vi "Main.vi"(0 "VI to load":string(combo)="Latch boolean simulation", 5 "STOP":bool, 11 "Error In":errorcluster) -> (15 "Error Out":errorcluster)   [LabVIEW 2016, in "Subpanel.lvlib"]
doc: "Source VI to test subpanel"
uses:
  Subpanel.lvlib
  NumericControlValueCoercion.vi
  BooleanControl.vi
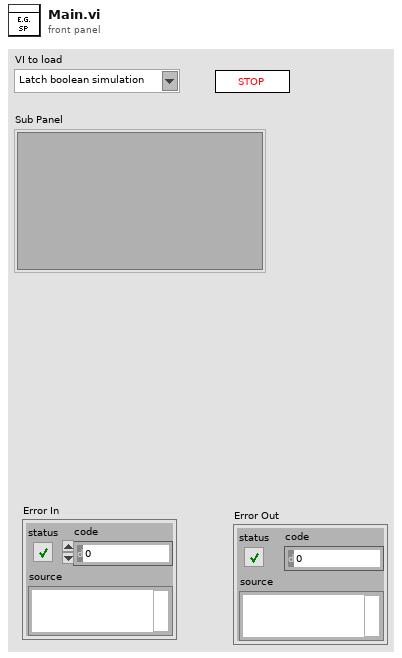
[diagram p1: front panel]
types:
  T1 = enum32{"Invalid", "Standard", "Closed", "Hidden", "Minimized", "Maximized"}
  T2 = enum32{"invalid app kind", "Development System", "Run Time System", "Student Edition", "Embedded LabVIEW", "Evaluation", "Custom"}
  T3 = cluster{"Core":cluster{"Current VI Reference":refnum<vi>, "Close Panel on Exit?":bool}, "Data Cluster":cluster{"Flags":cluster{"Source Code?":bool, "VI Inserted?":bool}, "VI Details":string[], "VI Ref[]":refnum<vi>[], "VI Ref":refnum<vi>}}
  T4 = cluster{"Flags":cluster{"Source Code?":bool, "VI Inserted?":bool}, "VI Details":string[], "VI Ref[]":refnum<vi>[], "VI Ref":refnum<vi>}
  T5 = cluster{"Current VI Reference":refnum<vi>, "Close Panel on Exit?":bool}
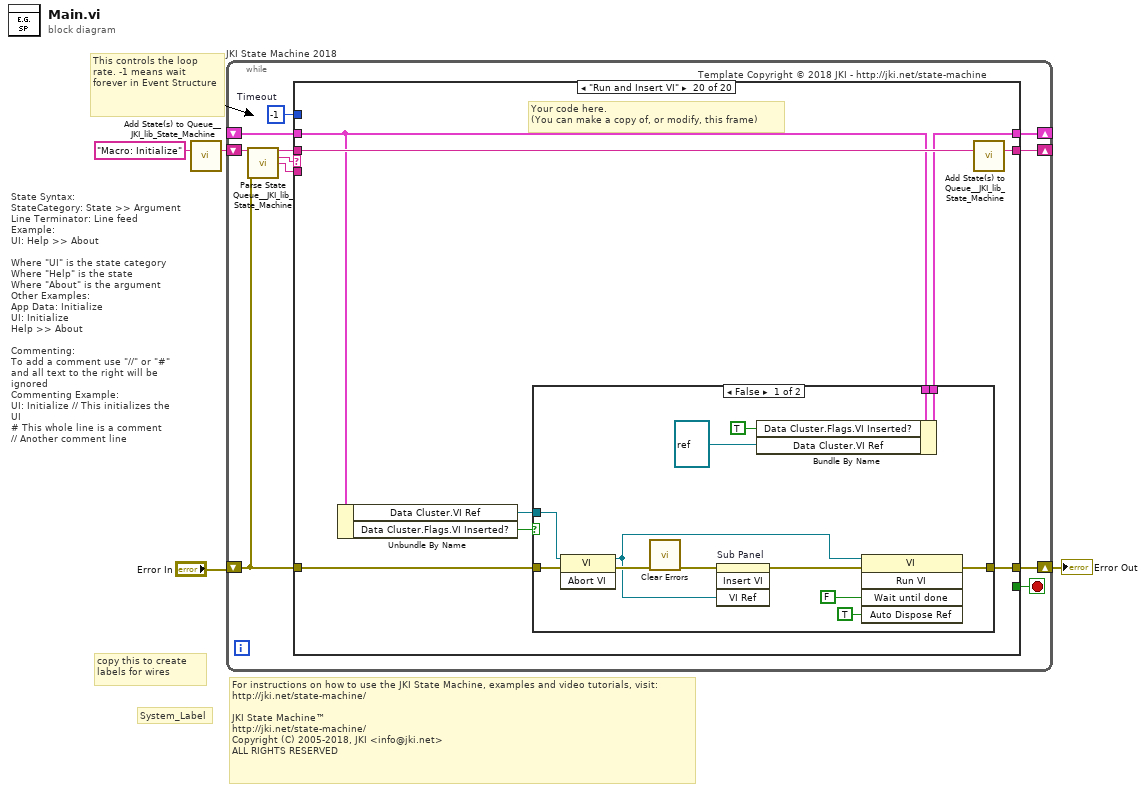
[diagram p0: block diagram]
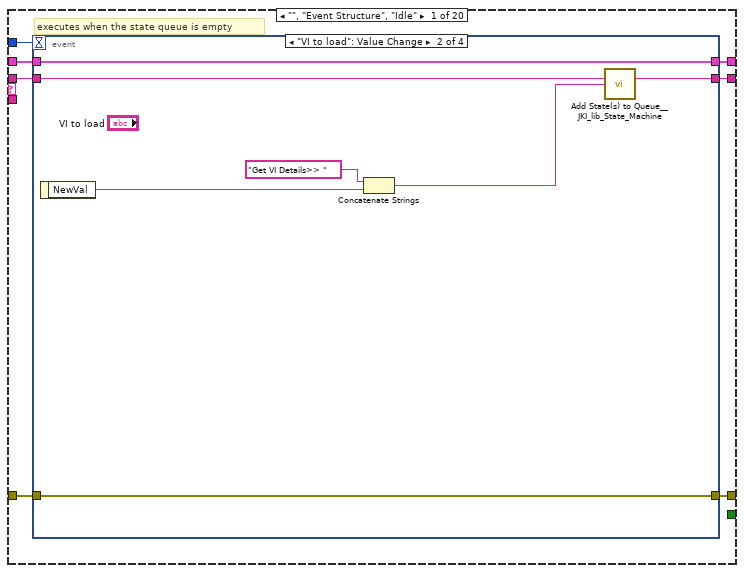
[diagram p2: hidden frame]
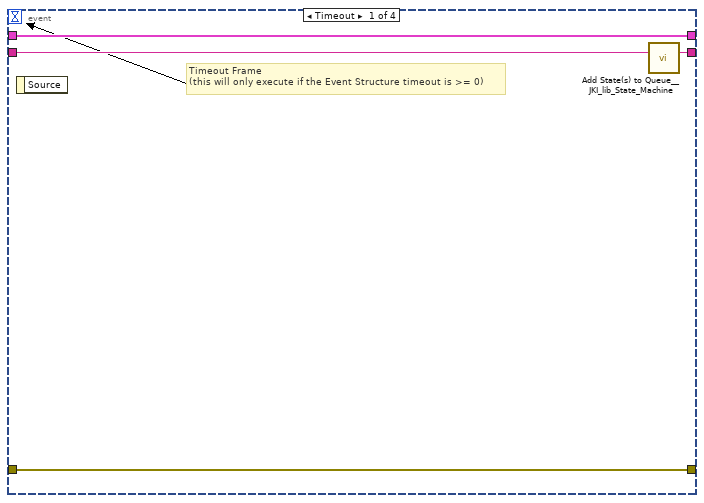
[diagram p3: hidden frame]
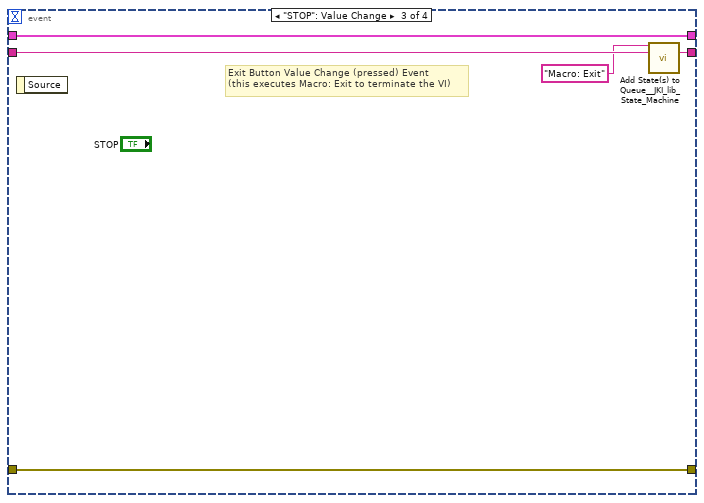
[diagram p4: hidden frame]
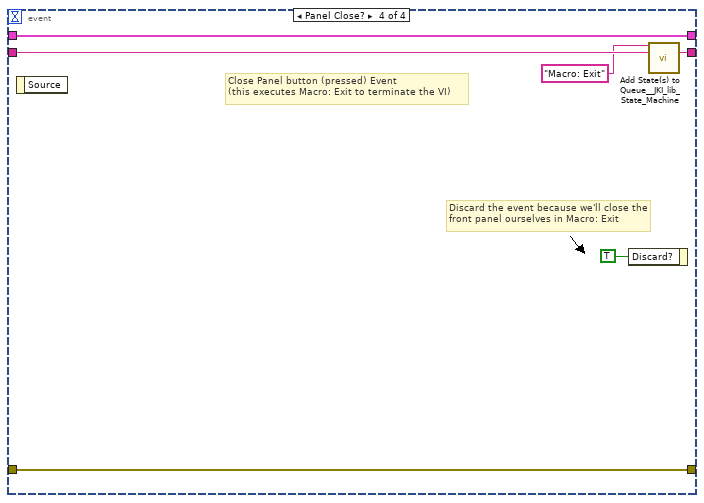
[diagram p5: hidden frame]
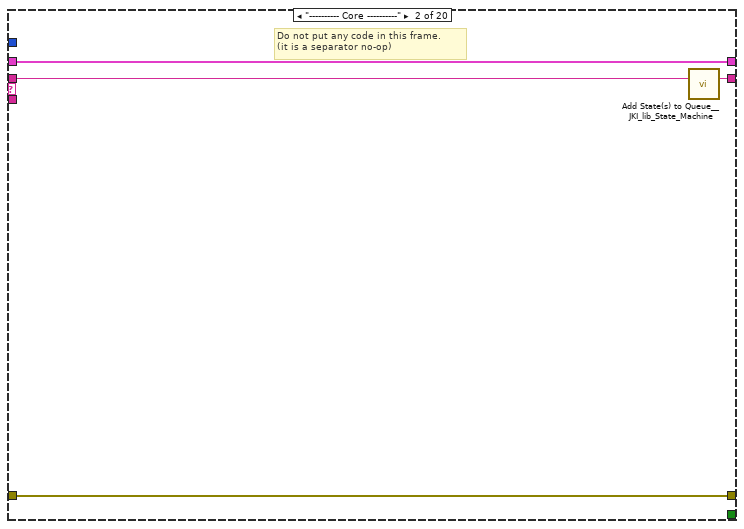
[diagram p6: hidden frame]
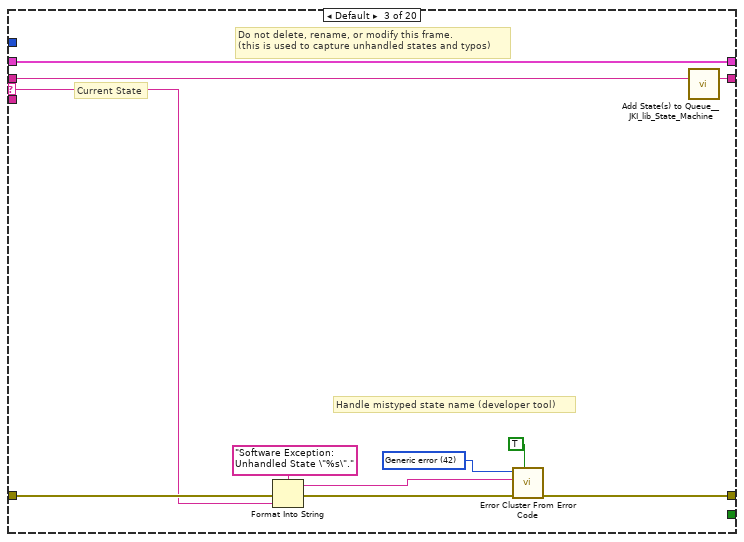
[diagram p7: hidden frame]
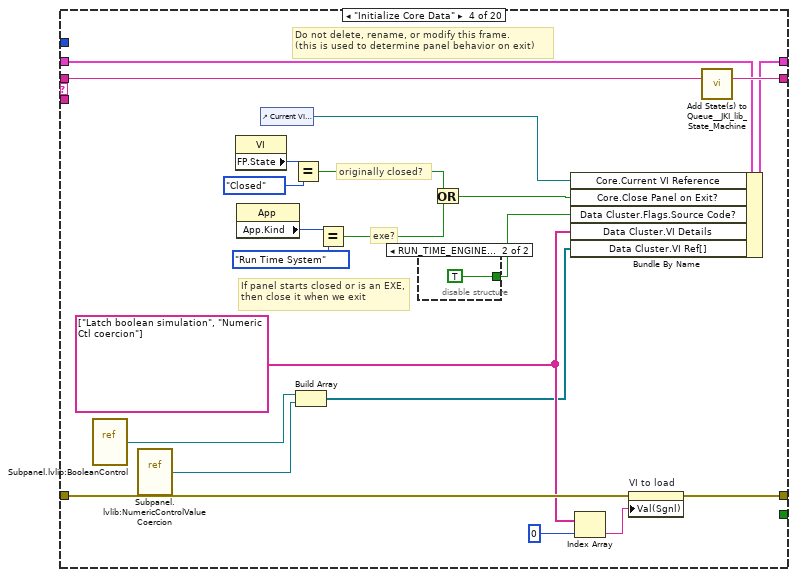
[diagram p8: hidden frame]
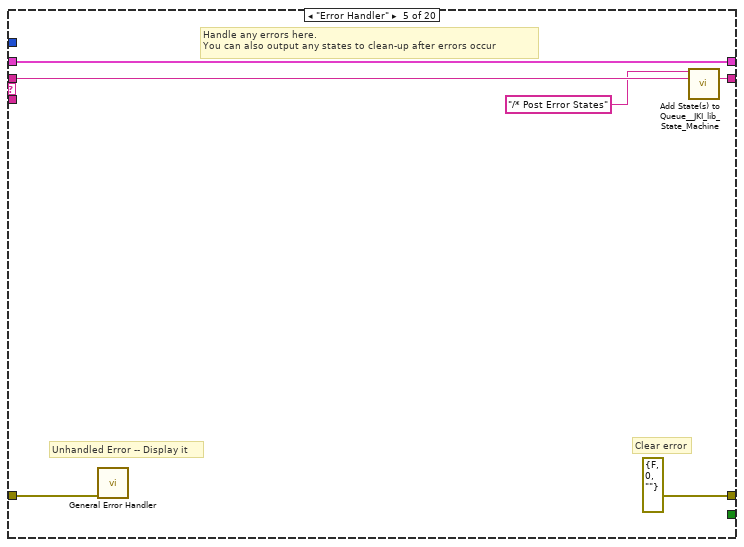
[diagram p10: hidden frame]
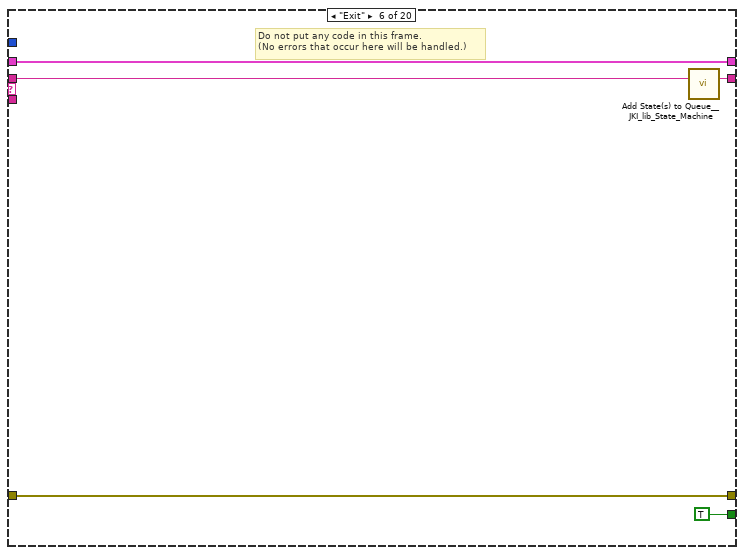
[diagram p11: hidden frame]
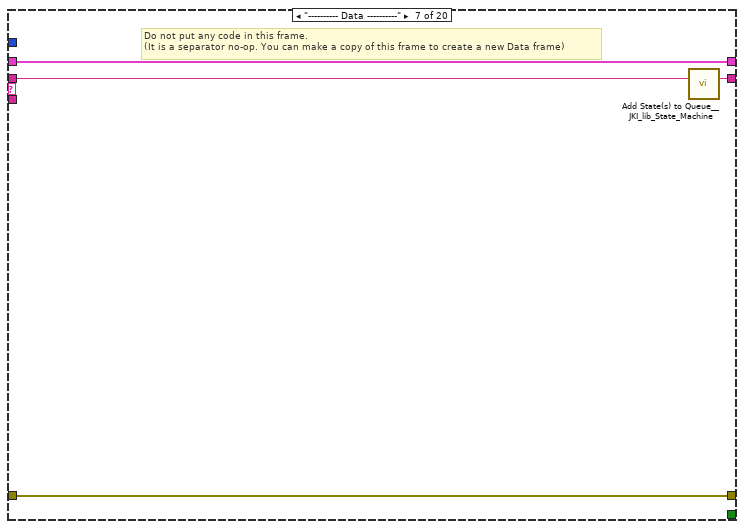
[diagram p12: hidden frame]
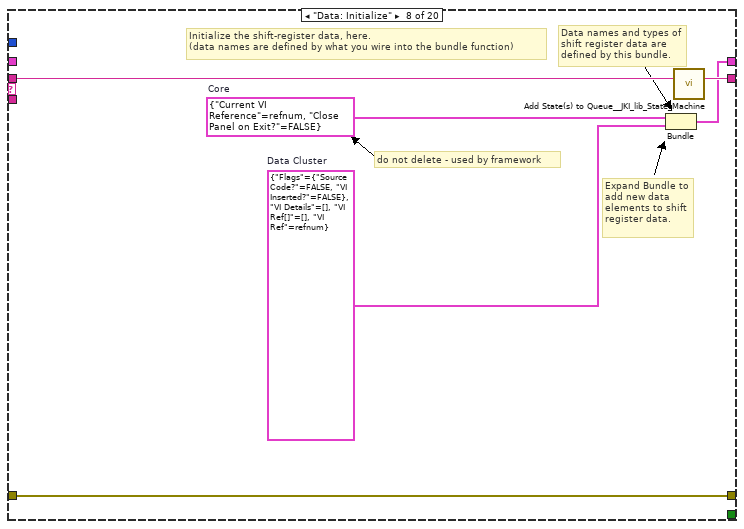
[diagram p13: hidden frame]
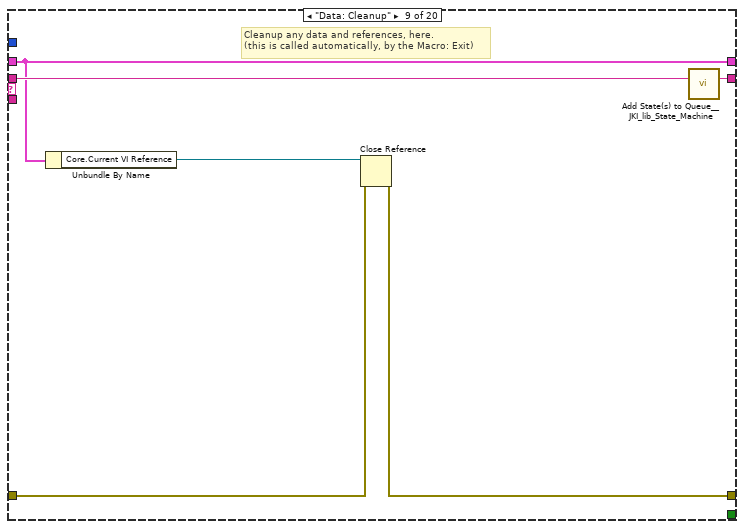
[diagram p14: hidden frame]
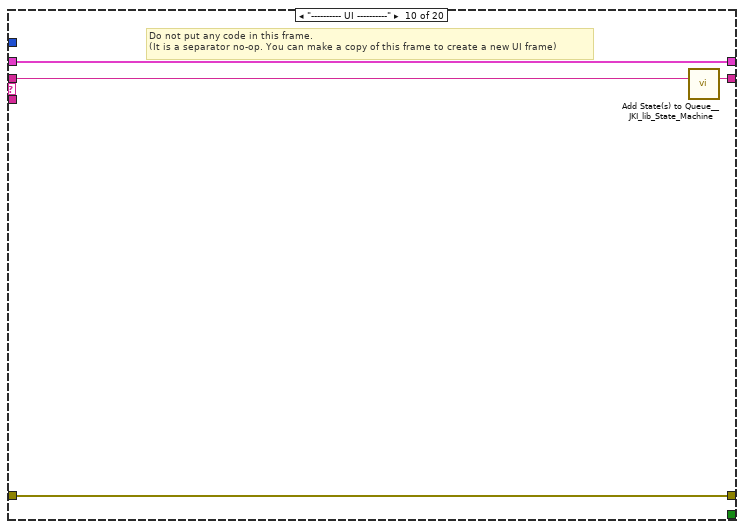
[diagram p15: hidden frame]
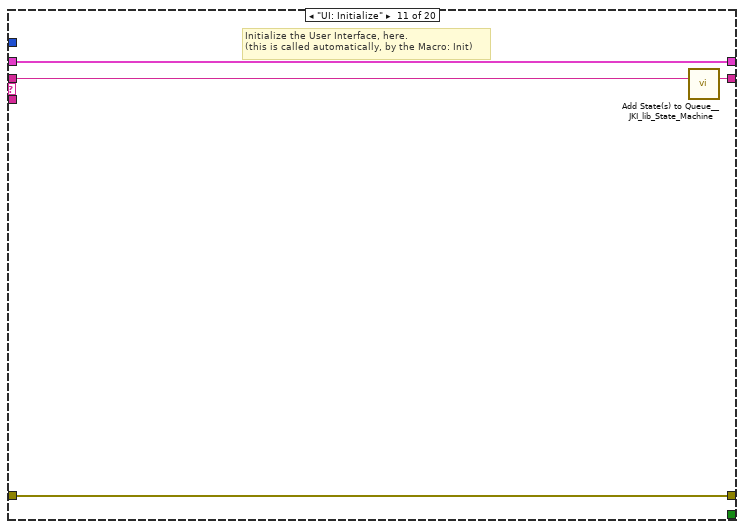
[diagram p16: hidden frame]
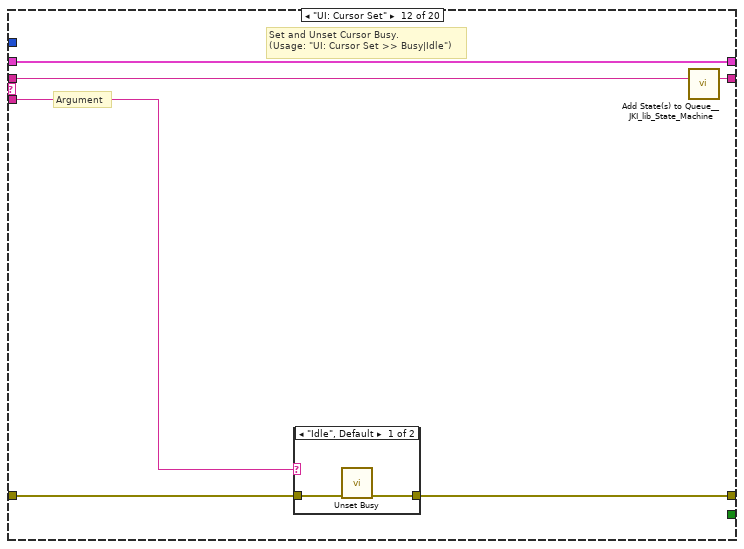
[diagram p17: hidden frame]
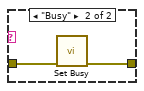
[diagram p18: hidden frame]
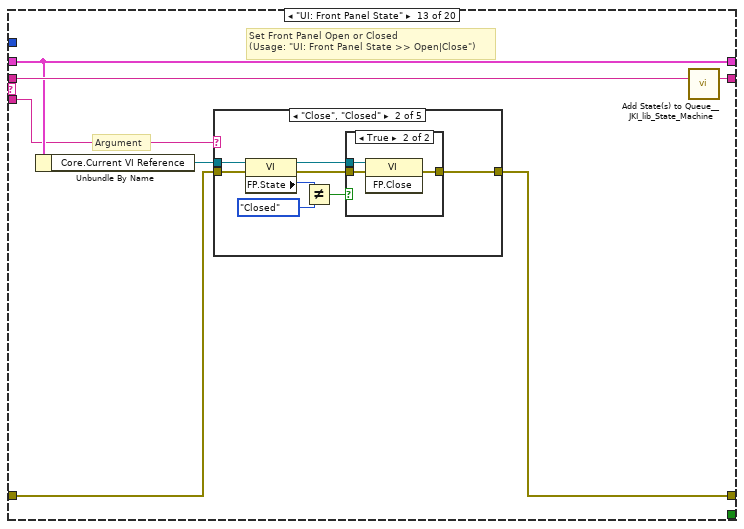
[diagram p19: hidden frame]
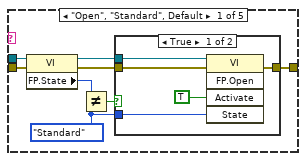
[diagram p20: hidden frame]
diagram:
  # "For instructions on how to use the JKI State Machine, examples and video tutorials, visit:\nhttp://jki.net/state-machine/\n\nJKI State Machine™\nhttp://jki.net/state-machine/\nCopyright (C) 2005-2018, JKI <info@jki.net>\nALL RIGHTS RESERVED"
  # "State Syntax:\nStateCategory: State >> Argument\nLine Terminator: Line feed\nExample:\nUI: Help >> About\n\nWhere \"UI\" is the state category\nWhere \"Help\" is the state\nWhere \"About\" is the argument\nOther Examples:\nApp Data: Initialize\nUI: Initialize\nHelp >> About\n\nCommenting:\nTo add a comment use \"//\" or \"#\" and all text to the right will be ignored\nCommenting Example:\nUI: Initialize // This initializes the UI\n# This whole line is a comment\n// Another comment line"
  # "copy this to create labels for wires"
  # "This controls the loop rate. -1 means wait forever in Event Structure"
  # "System_Label"
  n1 = call <vilib>:"Add State(s) to Queue__JKI_lib_State_Machine.vi"("State(s) in (\"\")"="Macro: Initialize") -> ("States Out"=w4:string)  [unwired: 14 in]
  n2 = while "JKI State Machine 2018" {
    shift-right: [w8] -> _
    shift-left: _ -> [w7]
    shift-right: [w11] -> w2
    shift-left: "Error In" -> [w5]
    shift-right: [w10] -> _
    shift-left: w4 -> [w12]
    stop <- w9 stop-if-true
    w6 = -1  # Timeout
    # "Template Copyright © 2018 JKI - http://jki.net/state-machine"
    n3 = call <vilib>:"Parse State Queue__JKI_lib_State_Machine.vi"("State Queue"=w12, "Error In (no error)"=w5) -> ("Remaining States"=w14:string, "Current State"=w15:string, "Arguments"=w13:string)  [unwired: 11 in]
    n4 = case shown="\"Run and Insert VI\"" w15 {
      selector: w15 -> [_ _ w49 _ _ _ _ _ _ _ _ _ _ _ _ _ _ _ _ _]
      tunnel: w14 -> [w22 w48 w53 w80 w87 w92 w96 w102 w108 w112 w116 w122 w133 w202 w207 w217 w221 w232 w240 w260]
      tunnel: w13 -> [_ _ _ _ _ _ _ _ _ _ _ w117 w127 _ _ _ _ w229 _ _]
      tunnel: w7 -> [w20 w45 w51 w73 w84 w90 w93 _ w103 w109 w114 w120 w129 w199 w204 w214 w218 w227 w234 w253]
      tunnel: [w19 w46 w55 w66 errorcluster {"status"=FALSE, "code"=0, "source"=""} ("error out") w89 w94 w99 w104 w110 w113 w118 w130 w200 w205 w215 w219 w223 w235 w255] -> w11
      tunnel: w5 -> [w18 w46 w54 w77 w83 w89 w94 w99 w105 w110 w113 w119 w131 w200 w205 w215 w219 w223 w236 w256]
      tunnel: [w21 w47 w52 w79 w86 w91 w95 w101 w107 w111 w115 w121 w132 w201 w206 w216 w220 w231 w239 w259] -> w10
      tunnel: [_ _ _ _ _ TRUE _ _ _ _ _ _ _ _ _ _ _ _ _ _] -> w9
      tunnel: [w17 w45 w51 w78 w84 w90 w93 w100 w103 w109 w114 w120 w129 w199 w204 w214 w218 w226 w233 w254] -> w8
      tunnel: w6 -> [w16 _ _ _ _ _ _ _ _ _ _ _ _ _ _ _ _ _ _ _]
      frame "", "Event Structure", "Idle" {
        # "executes when the state queue is empty"
        n5 = event shown="[1] \"VI to load\": Value Change" {
          selector: _ -> [_ _ _ _]
          dyn-events: _ -> [_ _ _ _]
          timeout: w16 -> [_ _ _ _]
          tunnel: w22 -> [w26 w33 w38 w44]
          tunnel: [w25 w32 w37 w43] -> w21
          tunnel: w20 -> [w23 w31 w35 w41]
          tunnel: [w24 w27 w36 w42] -> w19
          tunnel: w18 -> [w24 w27 w36 w42]
          tunnel: [w23 w31 w35 w41] -> w17
          event Timeout {
            # "Timeout Frame\n(this will only execute if the Event Structure timeout is >= 0)"
            n6 = event-data() -> ()  [unwired: 1 in, 1 out]
            n7 = call <vilib>:"Add State(s) to Queue__JKI_lib_State_Machine.vi"("State(s) in (\"\")"=w26) -> ("States Out"=w25:string)  [unwired: 14 in]
          }
          event "VI to load": Value Change {
            n8 = event-data() -> ("NewVal"=w30:string)  [unwired: 1 in]
            n9 = Concatenate Strings("Get VI Details>> " ("Item to Add"), w30) -> (w28:string)
            n10 = call <vilib>:"Add State(s) to Queue__JKI_lib_State_Machine.vi"("State(s) in (\"\")"=w33, "State(s) at Back (\"\")"=w28) -> ("States Out"=w32:string)  [unwired: 13 in]
          }
          event "STOP": Value Change {
            # "Exit Button Value Change (pressed) Event\n(this executes Macro: Exit to terminate the VI)"
            n11 = event-data() -> ()  [unwired: 1 in, 1 out]
            n12 = call <vilib>:"Add State(s) to Queue__JKI_lib_State_Machine.vi"("State(s) in Front (\"\")"="Macro: Exit", "State(s) in (\"\")"=w38) -> ("States Out"=w37:string)  [unwired: 13 in]
          }
          event Panel Close? {
            # "Discard the event because we'll close the front panel ourselves in Macro: Exit"
            # "Close Panel button (pressed) Event\n(this executes Macro: Exit to terminate the VI)"
            n13 = event-data() -> ()  [unwired: 1 in, 1 out]
            n14 = event-data("Discard?"=TRUE) -> ()  [unwired: 1 in, 1 out]
            n15 = call <vilib>:"Add State(s) to Queue__JKI_lib_State_Machine.vi"("State(s) in Front (\"\")"="Macro: Exit", "State(s) in (\"\")"=w44) -> ("States Out"=w43:string)  [unwired: 13 in]
          }
        }
      }
      frame "---------- Core ----------" {
        # "Do not put any code in this frame.\n(it is a separator no-op)"
        n16 = call <vilib>:"Add State(s) to Queue__JKI_lib_State_Machine.vi"("State(s) in (\"\")"=w48) -> ("States Out"=w47:string)  [unwired: 14 in]
      }
      frame Default {
        w58 = 42 items=["No error", "Argument error", "Memory is full", "Out of zone", "End of file", "File already open", "Generic file I/O error", "File not found", "File permission error", "Disk is full", "Duplicate path", "Too many files open", "System feature not enabled", "Resource file not found", "Cannot add resource", "Resource not found", "Image not found", "Image memory error", "Pen does not exist", "Config type invalid", "Config token not found", "Config parse error", "Config memory error", "Bad external code format", "Bad external code offset", "External code not present", "Null window", "Destroy window error", "Null menu", "Print aborted", "Bad print record", "Print driver error", "Windows error during printing", "Memory error during printing", "Print dialog error", "Generic print error", "Invalid device refnum", "Device not found", "Device parameter error", "Device unit error", "Cannot open device", "Device call aborted", "Generic error", "Cancelled by user", "Object ID too low", "Object ID too high", "Object not in heap", "Unknown heap", "Unknown object (invalid DefProc)", "Unknown object (DefProc not in table)", "Message out of range", "Invalid (null) method", "Unknown message", "Manager call not supported", "Bad address", "Network operation in progress", "Network operation timed out", "Connection is busy", "Network attribute not supported", "Network error", "Address in use", "System out of memory", "Connection aborted", "Connection refused", "Not connected", "Already connected", "Connection closed", "Initialization error (interapplication manager)", "Bad occurrence", "Wait on unbound occurrence handler", "Occurrence queue overflow", "Datalog type conflict", "Unused", "Unrecognized type (interapplication manager)", "Memory corrupt", "Failed to make temporary DLL", "Old CIN version", "Drag socket not found", "Failed to load drop-object", "Failed to register OLE object", "Failed to release OLE object", "Format specifier type mismatch", "Unknown format specifier", "Too few format specifiers", "Too many format specifiers", "Scan failed", "Newer CIN version", "Error converting to variant", "Runtime menu error", "Password tampered", "Variant attribute not found", "Incompatible variant data type", "Event data is not available", "Event Store is not present", "Occurrence is not found", "Event Queue is not created", "Event info is not available", "Refnum passed is NULL", "Error retrieving Class GUID", "Error retrieving CoClass GUID", "Error retrieving TypeLib GUID.", "Bad built application magic bytes.", "Specific driver is different from the specific driver associated with the Logical Name.", "There is no session opened to the class driver.", "Max Error", "MAX - Error with config objects", "MAX - Error loading configuration", "MAX - Group not supported"]
        # "Current State"
        # "Do not delete, rename, or modify this frame.\n(this is used to capture unhandled states and typos)"
        # "Handle mistyped state name (developer tool)"
        n17 = Format Into String(format string="Software Exception: Unhandled State \"%s\"." ("message"), error in=w54, w49) -> (resulting string=w57:string, error out=w56:errorcluster)  [unwired: 1 in]
        n18 = call <vilib>:"Error Cluster From Error Code.vi"("show call chain? (False)"=TRUE, "error in (no error)"=w56, "error message (\"\")"=w57, "error code (0)"=w58) -> ("error out"=w55:errorcluster)  [unwired: 5 in]
        n19 = call <vilib>:"Add State(s) to Queue__JKI_lib_State_Machine.vi"("State(s) in (\"\")"=w53) -> ("States Out"=w52:string)  [unwired: 14 in]
      }
      frame "Initialize Core Data" {
        w65 = string[] ["Latch boolean simulation", "Numeric Ctl coercion"]
        # "Do not delete, rename, or modify this frame.\n(this is used to determine panel behavior on exit)"
        # "originally closed?"
        # "exe?"
        # "If panel starts closed or is an EXE, then close it when we exit"
        n20 = vi-ref "Subpanel.lvlib:BooleanControl.vi"() -> (w61:refnum<vi>)
        n21 = vi-ref "Subpanel.lvlib:NumericControlValueCoercion.vi"() -> (w62:refnum<vi>)
        n22 = property class="VI"() -> ("FP.State"=w70:T1)  [unwired: 2 in, 2 out]
        n23 = property class="App"() -> ("App.Kind"=w76:T2)  [unwired: 2 in, 2 out]
        n24 = control-ref of="Current VI Reference"() -> (w71:refnum<vi>)
        n25 = Equal?(x=w70, y=T1."Closed" ("Front Panel Window:State")) -> (x = y?=w68:bool)
        n26 = Build Array(w61, w62) -> (w60:refnum<vi>[])
        n27 = Equal?(x=w76, y=T2."Run Time System" ("Application:Kind")) -> (x = y?=w74:bool)
        n28 = disable-structure shown="RUN_TIME_ENGINE==False" {
          disable-tunnel: [_ TRUE] -> w67
          frame condition #0 {
          }
          frame condition #1 (active) {
          }
        }
        n29 = Or(x=w68, y=w74) -> (x .or. y?=w72:bool)
        n30 = Bundle By Name(cluster=w73, "Core.Current VI Reference"=w71, "Core.Close Panel on Exit?"=w72, "Data Cluster.Flags.Source Code?"=w67, "Data Cluster.VI Details"=w65, "Data Cluster.VI Ref[]"=w60) -> (w78:T3)
        n31 = Index Array(array=w65, index=0 ("index (row)")) -> (element=w64:string)
        n32 = property on="VI to load" class="CmbBox"(error in=w77, "Val(Sgnl)"=w64) -> (error out=w66:errorcluster)  [unwired: 1 in, 1 out]
        n33 = call <vilib>:"Add State(s) to Queue__JKI_lib_State_Machine.vi"("State(s) in (\"\")"=w80) -> ("States Out"=w79:string)  [unwired: 14 in]
      }
      frame "Error Handler" {
        # "Unhandled Error -- Display it"
        # "Handle any errors here.\nYou can also output any states to clean-up after errors occur"
        # "Clear error"
        n34 = call <vilib>:"General Error Handler.vi"("error in (no error)"=w83) -> ()  [unwired: 10 in, 5 out]
        n35 = call <vilib>:"Add State(s) to Queue__JKI_lib_State_Machine.vi"("State(s) in Front (\"\")"="/* Post Error States", "State(s) in (\"\")"=w87) -> ("States Out"=w86:string)  [unwired: 13 in]
      }
      frame "Exit" {
        # "Do not put any code in this frame.\n(No errors that occur here will be handled.)"
        n36 = call <vilib>:"Add State(s) to Queue__JKI_lib_State_Machine.vi"("State(s) in (\"\")"=w92) -> ("States Out"=w91:string)  [unwired: 14 in]
      }
      frame "---------- Data ----------" {
        # "Do not put any code in this frame.\n(It is a separator no-op. You can make a copy of this frame to create a new Data frame)"
        n37 = call <vilib>:"Add State(s) to Queue__JKI_lib_State_Machine.vi"("State(s) in (\"\")"=w96) -> ("States Out"=w95:string)  [unwired: 14 in]
      }
      frame "Data: Initialize" {
        w97 = T4 {"Flags"={"Source Code?"=FALSE, "VI Inserted?"=FALSE}, "VI Details"=[], "VI Ref[]"=[], "VI Ref"=refnum}  # Data Cluster
        w98 = T5 {"Current VI Reference"=refnum, "Close Panel on Exit?"=FALSE}  # Core
        # "do not delete - used by framework"
        # "Expand Bundle to add new data elements to shift register data."
        # "Data names and types of shift register data are defined by this bundle."
        # "Initialize the shift-register data, here.\n(data names are defined by what you wire into the bundle function)"
        n38 = Bundle("Core"=w98, "Data Cluster"=w97) -> (w100:T3)  [unwired: 1 in]
        n39 = call <vilib>:"Add State(s) to Queue__JKI_lib_State_Machine.vi"("State(s) in (\"\")"=w102) -> ("States Out"=w101:string)  [unwired: 14 in]
      }
      frame "Data: Cleanup" {
        # "Cleanup any data and references, here.\n(this is called automatically, by the Macro: Exit)"
        n40 = Unbundle By Name(w103) -> ("Core.Current VI Reference"=w106:refnum<vi>)
        n41 = Close Reference(reference=w106, error in (no error)=w105) -> (error out=w104:errorcluster)
        n42 = call <vilib>:"Add State(s) to Queue__JKI_lib_State_Machine.vi"("State(s) in (\"\")"=w108) -> ("States Out"=w107:string)  [unwired: 14 in]
      }
      frame "---------- UI ----------" {
        # "Do not put any code in this frame.\n(It is a separator no-op. You can make a copy of this frame to create a new UI frame)"
        n43 = call <vilib>:"Add State(s) to Queue__JKI_lib_State_Machine.vi"("State(s) in (\"\")"=w112) -> ("States Out"=w111:string)  [unwired: 14 in]
      }
      frame "UI: Initialize" {
        # "Initialize the User Interface, here.\n(this is called automatically, by the Macro: Init)"
        n44 = call <vilib>:"Add State(s) to Queue__JKI_lib_State_Machine.vi"("State(s) in (\"\")"=w116) -> ("States Out"=w115:string)  [unwired: 14 in]
      }
      frame "UI: Cursor Set" {
        # "Argument"
        # "Set and Unset Cursor Busy.\n(Usage: \"UI: Cursor Set >> Busy|Idle\")"
        n45 = case shown="\"Idle\", Default" w117 {
          tunnel: w119 -> [w124 w126]
          tunnel: [w123 w125] -> w118
          frame "Idle", Default {
            n46 = call <vilib>:"Unset Busy.vi"("error in (no error)"=w124) -> ("error out"=w123:errorcluster)  [unwired: 10 in]
          }
          frame "Busy" {
            n47 = call <vilib>:"Set Busy.vi"("error in (no error)"=w126) -> ("error out"=w125:errorcluster)  [unwired: 9 in, 1 out]
          }
        }
        n48 = call <vilib>:"Add State(s) to Queue__JKI_lib_State_Machine.vi"("State(s) in (\"\")"=w122) -> ("States Out"=w121:string)  [unwired: 14 in]
      }
      frame "UI: Front Panel State" {
        # "Argument"
        # "Set Front Panel Open or Closed\n(Usage: \"UI: Front Panel State >> Open|Close\")"
        n49 = Unbundle By Name(w129) -> ("Core.Current VI Reference"=w128:refnum<vi>)
        n50 = case shown="\"Close\", \"Closed\"" w127 {
          tunnel: w131 -> [w139 w154 w165 w178 w191]
          tunnel: [w141 w155 w167 w180 w193] -> w130
          tunnel: w128 -> [w140 w152 w166 w179 w192]
          frame "Open", "Standard", Default {
            w134 = T1."Standard" ("State")
            n51 = property class="VI"(reference=w140, error in=w139) -> (reference out=w137:refnum<vi>, error out=w138:errorcluster, "FP.State"=w136:T1)
            n52 = Not Equal?(x=w136, y=w134) -> (x != y?=w135:bool)
            n53 = case shown="True" w135 {
              tunnel: [w145 w147] -> w141
              tunnel: w138 -> [w144 w147]
              tunnel: w137 -> [w143 _]
              tunnel: w134 -> [w142 _]
              frame True {
                n54 = invoke class="VI" method="FP.Open"(reference=w143, error in=w144, "Activate"=TRUE, "State"=w142) -> (error out=w145:errorcluster)  [unwired: 1 in, 4 out]
              }
              frame False {
              }
            }
          }
          frame "Close", "Closed" {
            n55 = property class="VI"(reference=w152, error in=w154) -> (reference out=w151:refnum<vi>, error out=w153:errorcluster, "FP.State"=w149:T1)
            n56 = Not Equal?(x=w149, y=T1."Closed" ("Front Panel Window:State")) -> (x != y?=w148:bool)
            n57 = case shown="True" w148 {
              tunnel: [w156 w159] -> w155
              tunnel: w153 -> [w156 w158]
              tunnel: w151 -> [_ w157]
              frame False {
              }
              frame True {
                n58 = invoke class="VI" method="FP.Close"(reference=w157, error in=w158) -> (error out=w159:errorcluster)  [unwired: 1 in, 2 out]
              }
            }
          }
          frame "Hidden", "Hide" {
            w160 = T1."Hidden" ("State")
            n59 = property class="VI"(reference=w166, error in=w165) -> (reference out=w163:refnum<vi>, error out=w164:errorcluster, "FP.State"=w162:T1)
            n60 = Not Equal?(x=w162, y=w160) -> (x != y?=w161:bool)
            n61 = case shown="True" w161 {
              tunnel: [w171 w172] -> w167
              tunnel: w164 -> [w170 w172]
              tunnel: w163 -> [w169 _]
              tunnel: w160 -> [w168 _]
              frame True {
                n62 = invoke class="VI" method="FP.Open"(reference=w169, error in=w170, "State"=w168) -> (error out=w171:errorcluster)  [unwired: 2 in, 4 out]
              }
              frame False {
              }
            }
          }
          frame "Minimize", "Minimized" {
            w173 = T1."Minimized" ("State")
            n63 = property class="VI"(reference=w179, error in=w178) -> (reference out=w176:refnum<vi>, error out=w177:errorcluster, "FP.State"=w175:T1)
            n64 = Not Equal?(x=w175, y=w173) -> (x != y?=w174:bool)
            n65 = case shown="True" w174 {
              tunnel: [w184 w185] -> w180
              tunnel: w177 -> [w183 w185]
              tunnel: w176 -> [w182 _]
              tunnel: w173 -> [w181 _]
              frame True {
                n66 = invoke class="VI" method="FP.Open"(reference=w182, error in=w183, "State"=w181) -> (error out=w184:errorcluster)  [unwired: 2 in, 4 out]
              }
              frame False {
              }
            }
          }
          frame "Maximize", "Maximized" {
            w186 = T1."Maximized" ("State")
            n67 = property class="VI"(reference=w192, error in=w191) -> (reference out=w189:refnum<vi>, error out=w190:errorcluster, "FP.State"=w188:T1)
            n68 = Not Equal?(x=w188, y=w186) -> (x != y?=w187:bool)
            n69 = case shown="True" w187 {
              tunnel: [w197 w198] -> w193
              tunnel: w190 -> [w196 w198]
              tunnel: w189 -> [w195 _]
              tunnel: w186 -> [w194 _]
              frame True {
                n70 = invoke class="VI" method="FP.Open"(reference=w195, error in=w196, "State"=w194) -> (error out=w197:errorcluster)  [unwired: 2 in, 4 out]
              }
              frame False {
              }
            }
          }
        }
        n71 = call <vilib>:"Add State(s) to Queue__JKI_lib_State_Machine.vi"("State(s) in (\"\")"=w133) -> ("States Out"=w132:string)  [unwired: 14 in]
      }
      frame "---------- Macro ----------" {
        # "Do not put any code in this frame.\n(It is a separator no-op. You can make a copy of this frame to create a new Macro frame)"
        n72 = call <vilib>:"Add State(s) to Queue__JKI_lib_State_Machine.vi"("State(s) in (\"\")"=w202) -> ("States Out"=w201:string)  [unwired: 14 in]
      }
      frame "Macro: Initialize" {
        w203 = "Data: Initialize\nInitialize Core Data\nUI: Initialize\nUI: Front Panel State >> Open"  # Data: Initialize Initialize Core Data UI: Initialize UI: Front Panel State >> Open
        # "Initialization Macro\n(This is called once, when the VI starts)"
        n73 = call <vilib>:"Add State(s) to Queue__JKI_lib_State_Machine.vi"("State(s) in Front (\"\")"=w203, "State(s) in (\"\")"=w207) -> ("States Out"=w206:string)  [unwired: 13 in]
      }
      frame "Macro: Exit" {
        # "Exit Macro\n(This is called once, when the VI exits)"
        n74 = Unbundle By Name(w214) -> ("Core.Close Panel on Exit?"=w213:bool)
        n75 = Select(t="UI: Front Panel State >> Close", s=w213, f="") -> (s? t:f=w210:string)
        n76 = call <vilib>:"Add State(s) to Queue__JKI_lib_State_Machine.vi"("State(s) in (\"\")"=w210, "State(s) at Back (\"\")"="Data: Cleanup\nRemove VI\nExit") -> ("States Out"=w208:string)  [unwired: 13 in]
        n77 = call <vilib>:"Add State(s) to Queue__JKI_lib_State_Machine.vi"("State(s) in Front (\"\")"=w208, "State(s) in (\"\")"=w217) -> ("States Out"=w216:string)  [unwired: 13 in]
      }
      frame "---------- Functions ----------" {
        # "Template Separator\n(You can make a copy of, or modify, this frame)"
        n78 = call <vilib>:"Add State(s) to Queue__JKI_lib_State_Machine.vi"("State(s) in (\"\")"=w221) -> ("States Out"=w220:string)  [unwired: 14 in]
      }
      frame "Get VI Details" {
        # "Your code here.\n(You can make a copy of, or modify, this frame)"
        n79 = Unbundle By Name(w227) -> ("Data Cluster.VI Ref[]"=w224:refnum<vi>[], "Data Cluster.VI Details"=w225:string[])
        n80 = Search 1D Array(1D array=w225, element=w229) -> (index of element=w230:i32)  [unwired: 1 in]
        n81 = Index Array(array=w224, index=w230) -> (element=w222:refnum<vi>)
        n82 = Bundle By Name(cluster=w227, "Data Cluster.VI Ref"=w222) -> (w226:T3)
        n83 = call <vilib>:"Add State(s) to Queue__JKI_lib_State_Machine.vi"("State(s) in (\"\")"=w232, "State(s) at Back (\"\")"="Remove VI\nRun and Insert VI" ("State(s) at Back (\"\")")) -> ("States Out"=w231:string)  [unwired: 13 in]
      }
      frame "Remove VI" {
        # "Your code here.\n(You can make a copy of, or modify, this frame)"
        n84 = Unbundle By Name(w234) -> ("Data Cluster.VI Ref"=w237:refnum<vi>, "Data Cluster.Flags.VI Inserted?"=w238:bool)
        n85 = case shown="True" w238 {
          tunnel: w236 -> [w242 w247]
          tunnel: [w242 w243] -> w235
          tunnel: w237 -> [_ _]
          tunnel: w234 -> [w241 w250]
          tunnel: [w241 w249] -> w233
          frame False {
          }
          frame True {
            n86 = invoke on="Sub Panel" class="SubPnl" method="Remove VI"(error in=w247) -> (error out=w246:errorcluster)  [unwired: 2 in, 2 out]
            n87 = call <vilib>:"Clear Errors.vi"("error in (no error)"=w246) -> ("error out"=w244:errorcluster)  [unwired: 5 in, 1 out]
            n88 = Bundle By Name(cluster=w250, "Data Cluster.Flags.VI Inserted?"=FALSE ("Flags.VI Inserted?")) -> (w249:T3)
            n89 = property on="Sub Panel" class="SubPnl"(error in=w244) -> (error out=w252:errorcluster, "InsertedVI"=w251:refnum<vi>)  [unwired: 1 in, 1 out]
            n90 = invoke class="VI" method="Abort VI"(reference=w251, error in=w252) -> (error out=w245:errorcluster)  [unwired: 1 in, 2 out]
            n91 = call <vilib>:"Clear Errors.vi"("error in (no error)"=w245) -> ("error out"=w243:errorcluster)  [unwired: 5 in, 1 out]
          }
        }
        n92 = call <vilib>:"Add State(s) to Queue__JKI_lib_State_Machine.vi"("State(s) in (\"\")"=w240) -> ("States Out"=w239:string)  [unwired: 14 in]
      }
      frame "Run and Insert VI" {
        # "Your code here.\n(You can make a copy of, or modify, this frame)"
        n93 = Unbundle By Name(w253) -> ("Data Cluster.VI Ref"=w258:refnum<vi>, "Data Cluster.Flags.VI Inserted?"=w257:bool)
        n94 = case shown="False" w257 {
          tunnel: w256 -> [w266 w274]
          tunnel: w258 -> [w264 _]
          tunnel: [w267 w274] -> w255
          tunnel: w253 -> [w271 w275]
          tunnel: [w270 w275] -> w254
          frame False {
            n95 = invoke class="VI" method="Abort VI"(reference=w264, error in=w266) -> (reference out=w263:refnum<vi>, error out=w265:errorcluster)  [unwired: 1 in, 1 out]
            n96 = call <vilib>:"Clear Errors.vi"("error in (no error)"=w265) -> ("error out"=w262:errorcluster)  [unwired: 5 in, 1 out]
            n97 = invoke on="Sub Panel" class="SubPnl" method="Insert VI"(error in=w262, "VI Ref"=w263) -> (error out=w268:errorcluster)  [unwired: 2 in, 3 out]
            n98 = Bundle By Name(cluster=w271, "Data Cluster.Flags.VI Inserted?"=TRUE ("Flags.VI Inserted?"), "Data Cluster.VI Ref"=refnum<vi> refnum ("VI Ref")) -> (w270:T3)
            n99 = invoke class="VI" method="Run VI"(reference=w263, error in=w268, "Wait until done"=FALSE ("Wait Until Done"), "Auto Dispose Ref"=TRUE ("Auto Dispose Reference")) -> (error out=w267:errorcluster)  [unwired: 1 in, 4 out]
          }
          frame True {
          }
        }
        n100 = call <vilib>:"Add State(s) to Queue__JKI_lib_State_Machine.vi"("State(s) in (\"\")"=w260) -> ("States Out"=w259:string)  [unwired: 14 in]
      }
    }
  }
  "Error Out" <- w2
